vi "NKTP_API_RegUserEvents.vi"(8 "error in":errorcluster) -> (0 "error out":errorcluster, 1 "Register Status User Event":refnum<user-event>, 2 "Device Status User Event":refnum<user-event>, 3 "Port Status User Event":refnum<user-event>, 5 "Event Registration Refnum":refnum<event-registration>)   [LabVIEW 2015, in "NKTP_API.lvlib"]
doc: "Registers LabVIEW User Events for Device, Port and Register callbacks from the NKTP.dll. \nYour own user events can be inserted into the UI event registration node as long as you make sure that they are registrated in alphabetical order."
uses:
  <instrlib>/NKTP_API/NKTP_API.lvlib
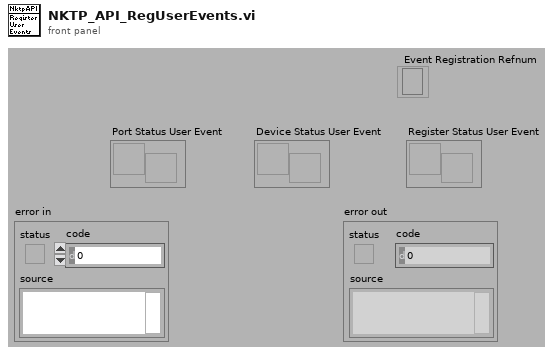
[diagram p1: front panel]
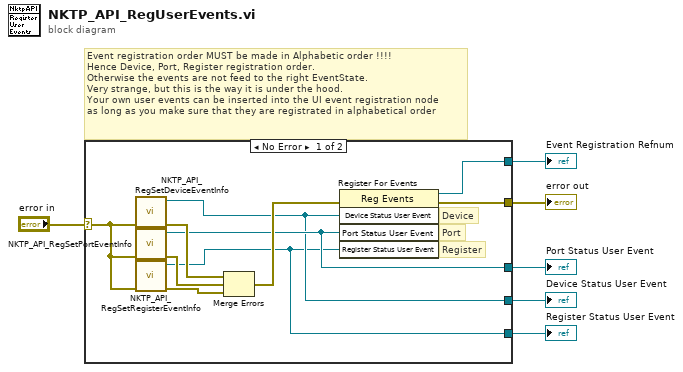
[diagram p0: block diagram]
diagram:
  # "Event registration order MUST be made in Alphabetic order !!!!\nHence Device, Port, Register registration order. \nOtherwise the events are not feed to the right EventState. \nVery strange, but this is the way it is under the hood.\nYour own user events can be inserted into the UI event registration node\nas long as you make sure that they are registrated in alphabetical order"
  n1 = case shown="No Error" "error in" {
    selector: "error in" -> [w14 w17]
    tunnel: [w9 _] -> w6
    tunnel: [w16 _] -> w2
    tunnel: [w8 _] -> w5
    tunnel: [w7 _] -> w4
    tunnel: [w10 w17] -> w3
    frame No Error {
      # "Register"
      # "Port"
      # "Device"
      n2 = call <instrlib>:"NKTP_API_RegSetDeviceEventInfo.vi"("error in"=w14) -> ("error out"=w11:errorcluster, "Device Status User Event"=w8:refnum<user-event>)  [unwired: 9 in]
      n3 = call <instrlib>:"NKTP_API_RegSetPortEventInfo.vi"("error in"=w14) -> ("error out"=w12:errorcluster, "Port Status User Event"=w9:refnum<user-event>)  [unwired: 9 in]
      n4 = call <instrlib>:"NKTP_API_RegSetRegisterEventInfo.vi"("error in"=w14) -> ("error out"=w13:errorcluster, "Register Status User Event"=w7:refnum<user-event>)  [unwired: 9 in]
      n5 = Merge Errors(w11, w12, w13) -> (w15:errorcluster)
      n6 = register-events(error in=w15, w8, w9, w7) -> (reference out=w16:refnum<event-registration>, error out=w10:errorcluster)  [unwired: 1 in]
    }
    frame Error {
    }
  }
  "error out" <- w3
  "Port Status User Event" <- w6
  "Device Status User Event" <- w5
  "Register Status User Event" <- w4
  "Event Registration Refnum" <- w2
